vi "Create Dispatcher.vi"(7 "FIFO Options":T1, 8 "error in (no error)":errorcluster, 10 "Plugins":refnum<class "Plugin.lvclass">[](array[class]), 11 "Framework in":refnum<class "Framework.lvclass">) -> (0 "error out":errorcluster, 2 "Dispatcher Thread":refnum<class "Dispatcher Thread.lvclass">, 3 "Framework out":refnum<class "Framework.lvclass">)   [LabVIEW 2017, in "DSF Core.lvlib" / "Framework.lvclass"]
uses:
  Framework.lvclass
  Plugin/Plugin.lvclass
  Dispatcher/Dispatcher Thread.lvclass
  Typedefs/FIFO Flags.ctl
  Thread/Thread Settings.ctl
  Framework.lvclass/Framework.ctl
  Thread/Thread.lvclass
  DSF Core.lvlib
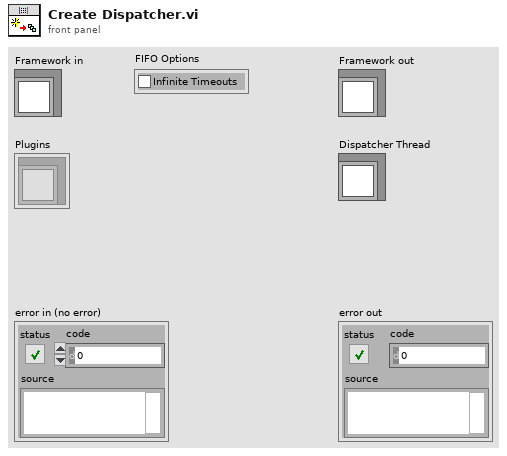
[diagram p1: front panel]
types:
  T1 = typedef "DSF Core.lvlib/FIFO Flags.ctl" = cluster{"Infinite Timeouts":bool}
  T2 = typedef "DSF Core.lvlib/Thread.lvclass/Thread Settings.ctl" = cluster{"Priority":u16, "Processor":i32, "ID":i32}
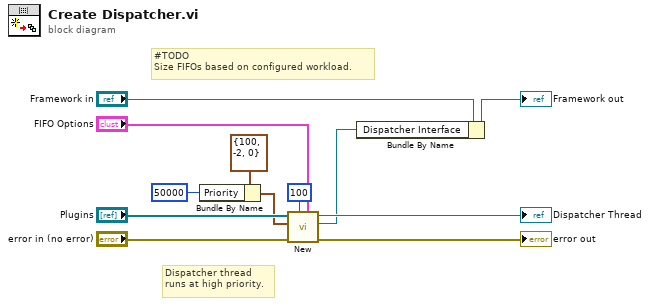
[diagram p0: block diagram]
diagram:
  # "Dispatcher thread runs at high priority."
  # "#TODO\nSize FIFOs based on configured workload."
  n1 = Bundle By Name(cluster=T2 {"Priority"=100, "Processor"=-2, "ID"=0} ("Thread Parameters"), "Priority"=u16 50000 ("priority (100)")) -> (w1:T2)
  n2 = call "New.vi"("FIFO Options"="FIFO Options", "fifo depths"=u32 100, "error in (no error)"="error in (no error)", "Thread Parameters"=w1, "Plugins"="Plugins") -> ("error out"=→"error out":errorcluster, "Dispatcher Interface"=w7:refnum<class "Dispatcher Interface.lvclass">, "Dispatcher Thread"=→"Dispatcher Thread":refnum<class "Dispatcher Thread.lvclass">)  [unwired: 4 in]
  n3 = Bundle By Name(cluster="Framework in", "Dispatcher Interface"=w7) -> (→"Framework out":refnum<class "Framework.lvclass">)
